vi "ThreeWaySwitch.vi"(0 "Sync1":bool, 1 "Sync0":bool, 2 "Sync2":bool, 3 "Sync0 last state":bool, 4 "Sync2 last state":bool, 5 "Sync1 last state":bool) -> (6 "Sync0out":bool, 7 "Sync1out":bool, 8 "Sync2out":bool)   [LabVIEW 2012]
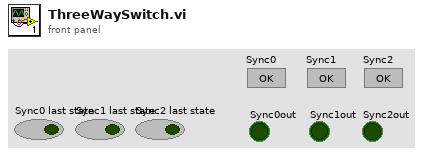
[diagram p1: front panel]
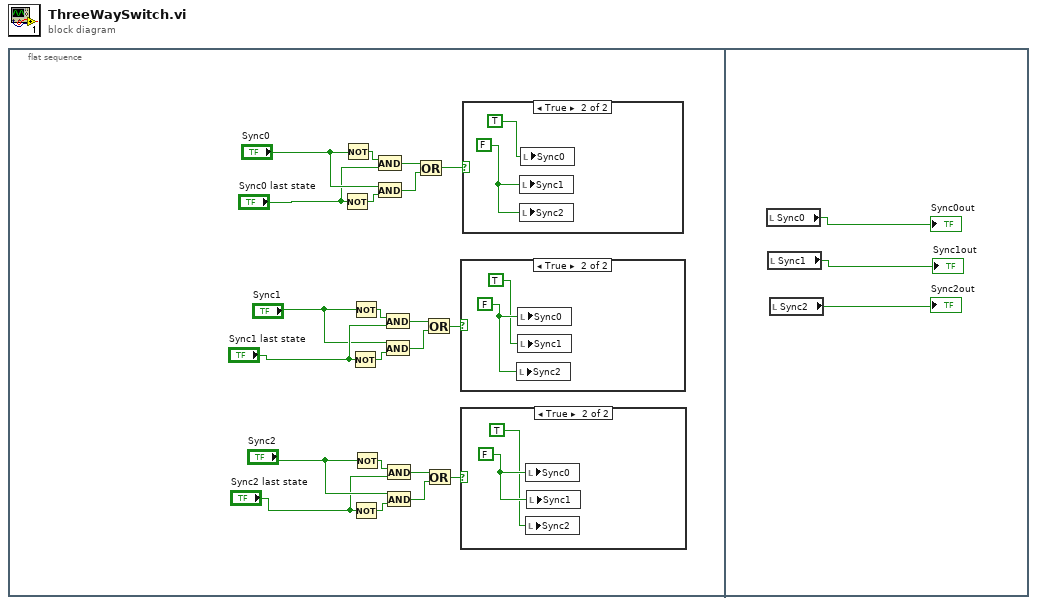
[diagram p0: block diagram]
diagram:
  n1 = flat-sequence {
    frame #0 {
      n2 = Not(x="Sync0 last state") -> (.not. x?=w21:bool)
      n3 = Not(x="Sync0") -> (.not. x?=w17:bool)
      n4 = Not(x="Sync1 last state") -> (.not. x?=w14:bool)
      n5 = Not(x="Sync1") -> (.not. x?=w11:bool)
      n6 = Not(x="Sync2 last state") -> (.not. x?=w10:bool)
      n7 = Not(x="Sync2") -> (.not. x?=w7:bool)
      n8 = And(x=w17, y="Sync0 last state") -> (x .and. y?=w18:bool)
      n9 = And(x="Sync0", y=w21) -> (x .and. y?=w19:bool)
      n10 = And(x=w11, y="Sync1 last state") -> (x .and. y?=w12:bool)
      n11 = And(x="Sync1", y=w14) -> (x .and. y?=w13:bool)
      n12 = And(x=w7, y="Sync2 last state") -> (x .and. y?=w8:bool)
      n13 = And(x="Sync2", y=w10) -> (x .and. y?=w9:bool)
      n14 = Or(x=w18, y=w19) -> (x .or. y?=w20:bool)
      n15 = Or(x=w12, y=w13) -> (x .or. y?=w5:bool)
      n16 = Or(x=w8, y=w9) -> (x .or. y?=w6:bool)
      n17 = case shown="True" w5 {
        frame False {
        }
        frame True {
          w25 = FALSE ("Sync1")
          n18 = local write "Sync2"(w25) -> ()
          n19 = local write "Sync0"(w25) -> ()
          n20 = local write "Sync1"(TRUE ("Sync0")) -> ()
        }
      }
      n21 = case shown="True" w6 {
        frame False {
        }
        frame True {
          w23 = FALSE ("Sync1")
          n22 = local write "Sync0"(w23) -> ()
          n23 = local write "Sync2"(TRUE ("Sync0")) -> ()
          n24 = local write "Sync1"(w23) -> ()
        }
      }
      n25 = case shown="True" w20 {
        frame False {
        }
        frame True {
          w27 = FALSE ("Sync1")
          n26 = local write "Sync1"(w27) -> ()
          n27 = local write "Sync2"(w27) -> ()
          n28 = local write "Sync0"(TRUE ("Sync0")) -> ()
        }
      }
    }
    frame #1 {
      n29 = local read "Sync0"() -> (→"Sync0out":bool)
      n30 = local read "Sync1"() -> (→"Sync1out":bool)
      n31 = local read "Sync2"() -> (→"Sync2out":bool)
    }
  }
